vi "get_line.vi"(8 "error in (no error)":errorcluster, 10 "line index":i32, 11 "PositionSignals in":refnum<class "PositionSignals.lvclass">) -> (0 "error out":errorcluster, 2 "pixel values":T1, 3 "PositionSignals out":refnum<class "PositionSignals.lvclass">)   [LabVIEW 2010, in "PositionSignals.lvclass"]
uses:
  PositionSignals.lvclass
  common/classes/ImageCollection/ImageCollection/pixel_positions_cluster.ctl
  common/classes/ImageCollection/ImageCollection/ImageCollection.lvclass
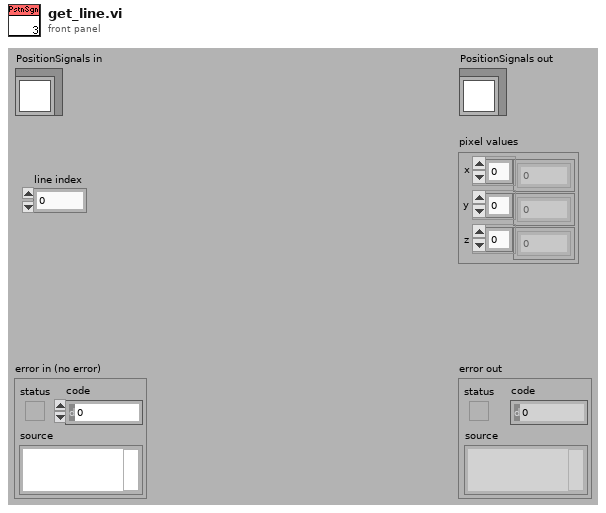
[diagram p1: front panel]
types:
  T1 = typedef "ImageCollection.lvclass/pixel_positions_cluster.ctl" = cluster{"x":dbl[], "y":dbl[], "z":dbl[]}
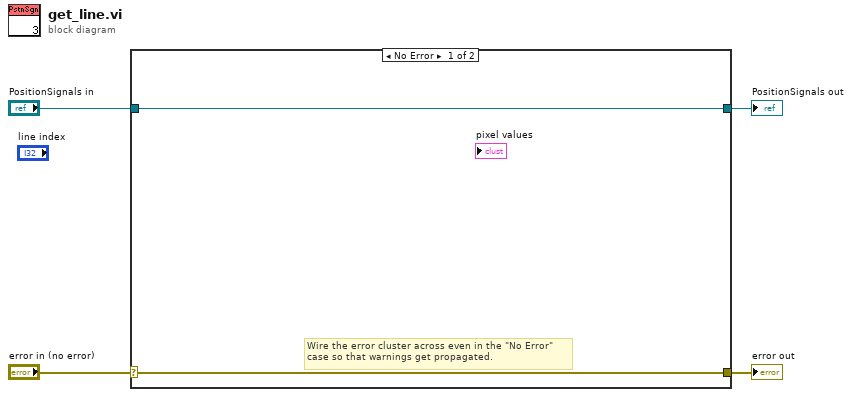
[diagram p0: block diagram]
diagram:
  n1 = case shown="No Error" "error in (no error)" {
    selector: "error in (no error)" -> [w5 w8]
    tunnel: [w5 w8] -> w3
    tunnel: [w6 w7] -> w1
    tunnel: "PositionSignals in" -> [w6 w7]
    frame No Error {
      # "Wire the error cluster across even in the \"No Error\"\ncase so that warnings get propagated."
    }
    frame Error {
    }
  }
  "error out" <- w3
  "PositionSignals out" <- w1
